vi "HilbertLogCompress.vi"(11 "Array in":dbl[][](array[numeric])) -> (3 "Array out":dbl[][](array[numeric]))   [LabVIEW 2022 SP3]
uses:
  <vilib>/Analysis/NI_AALPro.lvlib
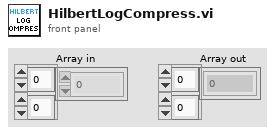
[diagram p1: front panel]
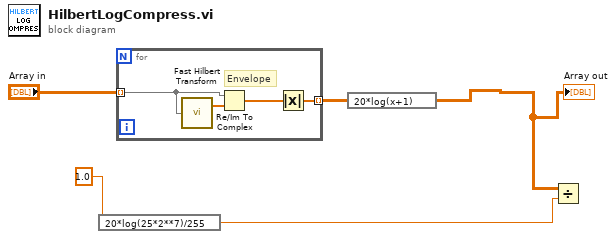
[diagram p0: block diagram]
diagram:
  n1 = expression code="20*log(25*2**7)/255"(sgl 1.0) -> (w2:sgl)
  n2 = for {
    tunnel: "Array in" -> [w7] mode=indexing
    tunnel: [w8] -> w4 mode=indexing
    # "Envelope"
    n3 = call <vilib>:"Fast Hilbert Transform.vi"("X"=w7) -> ("Hilbert{X}"=w6:dbl[])  [unwired: 1 out]
    n4 = Re/Im To Complex(1:w6, 2:w7) -> (0:w9:cdb[])
    n5 = Absolute Value(x=w9) -> (abs(x)=w8:dbl[])
  }
  n6 = expression code="20*log(x+1)"(w4) -> (w1:dbl[][])
  "Array out" <- w1
  n7 = Divide(x=w1, y=w2) -> ()  [unwired: 1 out]
